vi "MU Calibration Number Of Revolutions.vi"(8 "error in (no error)":errorcluster, 11 "AnalyzeResultHandle":T1) -> (0 "error out (no error)":errorcluster, 3 "NumberOfRevolutions":dbl)   [LabVIEW 2017, in "MU_3SL_interface.lvlib"]
uses:
  MU_3SL_interface.lvlib
  handles/CalibrationAnalyzeResultHandle.ctl
  lib/MU_3SL_interface.dll
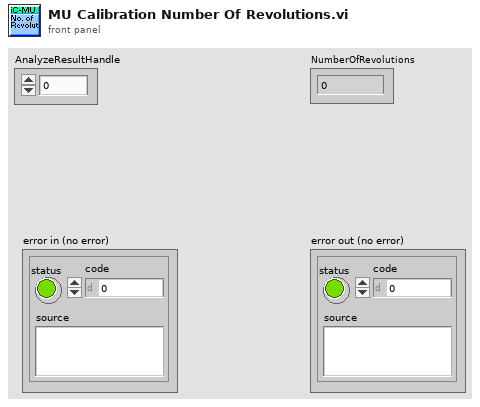
[diagram p1: front panel]
types:
  T1 = typedef "MU_3SL_interface.lvlib/CalibrationAnalyzeResultHandle.ctl" = u64
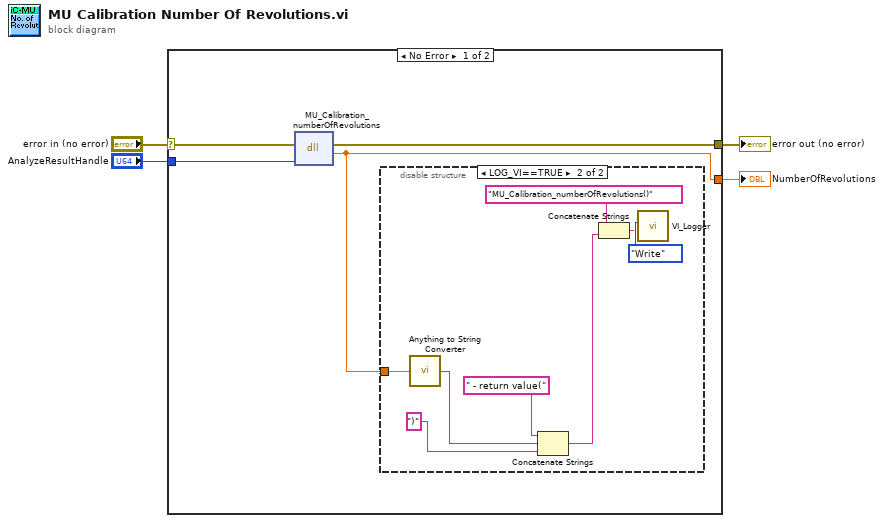
[diagram p0: block diagram]
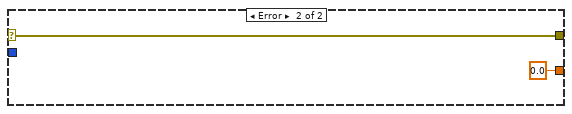
[diagram p3: hidden frame]
diagram:
  n1 = case shown="No Error" "error in (no error)" {
    selector: "error in (no error)" -> [w8 w18]
    tunnel: [w7 w18] -> w4
    tunnel: "AnalyzeResultHandle" -> [w6 _]
    tunnel: [w5 0.0 ("NumberOfRevolutions")] -> w1
    frame No Error {
      n2 = dll-call lib="C:/Users/bes/AppData/Roaming/work/mu_9so/icsubmodules/soft_mu_3sl_master/lv_interface/lib/MU_3SL_interface**.*" fn="MU_Calibration_numberOfRevolutions"(error in=w8, "AnalyzeResultHandle"=w6) -> (error out=w7:errorcluster, "NumberOfRevolutions"=w5:dbl)  [unwired: 3 in, 1 out]
      n3 = disable-structure shown="LOG_VI==TRUE" {
        disable-tunnel: w5 -> [_ w10]
        frame condition #0 {
        }
        frame condition #1 (active) {
          n4 = call "Anything to String Converter.vi"("anything"=w10) -> ("String"=w9:string)
          n5 = Concatenate Strings(" - return value(" ("string"), w9, ")" ("string")) -> (w11:string)
          n6 = Concatenate Strings("MU_Calibration_numberOfRevolutions()" ("Info in"), w11) -> (w14:string)
          n7 = call "VI_Logger.vi"("Action (Read)"=enum16{"Write", "Read"}."Write", "Info in"=w14) -> ()  [unwired: 8 in, 2 out]
        }
      }
    }
    frame Error {
    }
  }
  "error out (no error)" <- w4
  "NumberOfRevolutions" <- w1
